vi "Measurement UI.vi"() -> ()   [LabVIEW 2021, in "adc_linearityMeasurement.lvlib"]
uses:
  adc_linearityMeasurement.lvlib
panel:
  in  "MeasGraphs":T1(tab)
  out "TimeDomain":waveform(dbl)(graph) caption="AC"
  out "Histogram":T2(graph) caption="TimeDomain 2"
  out "DNL waveform":dbl[](graph) caption="AC"
  out "INL waveform":dbl[](graph) caption="AC"
  out "Channel name":string
  out "Number of missing codes":i32
  out "Minimum hits position":i32
  out "Minimum hits per code":i32
  out "INL position":i32
  out "INL":dbl
  out "DNL position":i32
  out "DNL":dbl
  out "Histogram: h(x)":i32[](array[numeric])
  out "Histogram X":dbl[](array[numeric])
  out "Time domain":dbl[](array[numeric])
  out "dt":dbl
  in  "Digital capture resource name":string
  in  "Analog source resource name":string
  out "MeasTable":string[][](table)
  in  "MeasSettingsOptions":i32(listbox)
  in  "Digital capture":string="Digital capture"
  in  "Analog source":string="Analog source"
  in  "ADC parameters":string="ADC parameters"
  in  "MeasSettings":bool
  out "Samples to acquire":u32 caption="SAMPLES TO ACQUIRE"
  in  "Digital capture test duration":dbl=800000.0 caption="TEST DURATION" format="%#_6ps"
  in  "Triangle frequency":dbl=20.0 caption="FREQUENCY" format="%#_6pHz"
  in  "Triangle amplitude":dbl=5.1 caption="AMPLITUDE" format="%#_6pV"
  in  "Sine amplitude":dbl=5.1 caption="AMPLITUDE" format="%#_6pV"
  in  "Sine frequency":dbl=1000.0 caption="FREQUENCY" format="%#_6pHz"
  out "Input frequency":dbl caption="INPUT FREQUENCY" format="%#_6pHz"
  in  "Input channel":i32 caption="INPUT CHANNEL" min=0 max=100 step=1
  in  "Ramp amplitude":dbl=5.05 caption="RAMP AMPLITUDE" format="%#_6pV"
  in  "Ramp type":u32(ring) caption="RAMP TYPE" items=["Ascending", "Descending"]
  in  "Ramp duration":dbl=10.0 caption="RAMP DURATION" format="%#_6ps"
  in  "Full scale range":dbl=10.0 caption="FULL SCALE RANGE" format="%#_6pV"
  in  "Input signal":u32(ring) caption="INPUT  SIGNAL" items=["Sine", "Triangle", "Ramp"]
  in  "Digital capture sample rate":dbl=800000.0 caption="SAMPLE RATE" format="%#_6pS/s"
  in  "DSGresourcename":tag caption="RESOURCE NAME"
  in  "DPIresourcename":refnum<k15> caption="RESOURCE NAME"
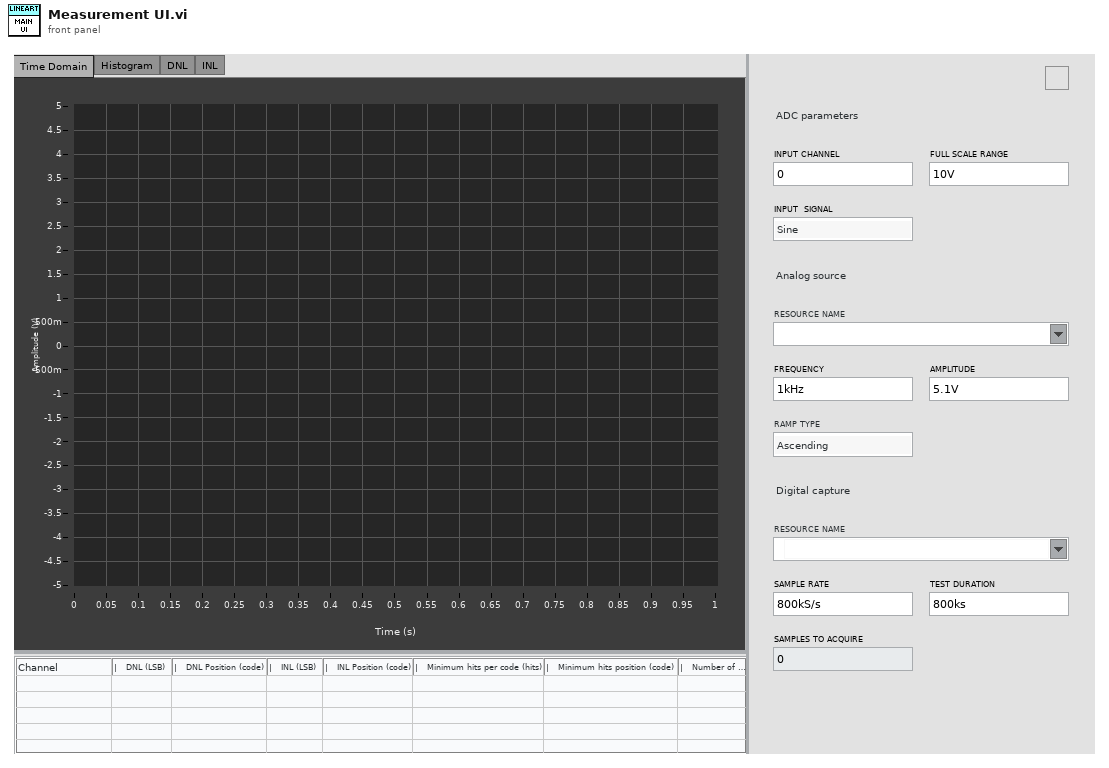
[diagram p1: front panel]
types:
  T1 = enum32{"Time Domain", "Histogram", "DNL", "INL", "Hiden controls"}
  T2 = cluster{"X Values":dbl[], "Histogram: h(x)":i32[]}
  T3 = enum16{"open", "replace", "create", "open or create", "replace or create", "replace or create with confirmation"}
  T4 = cluster{"Histogram X":dbl[], "Histogram: h(x)":i32[]}
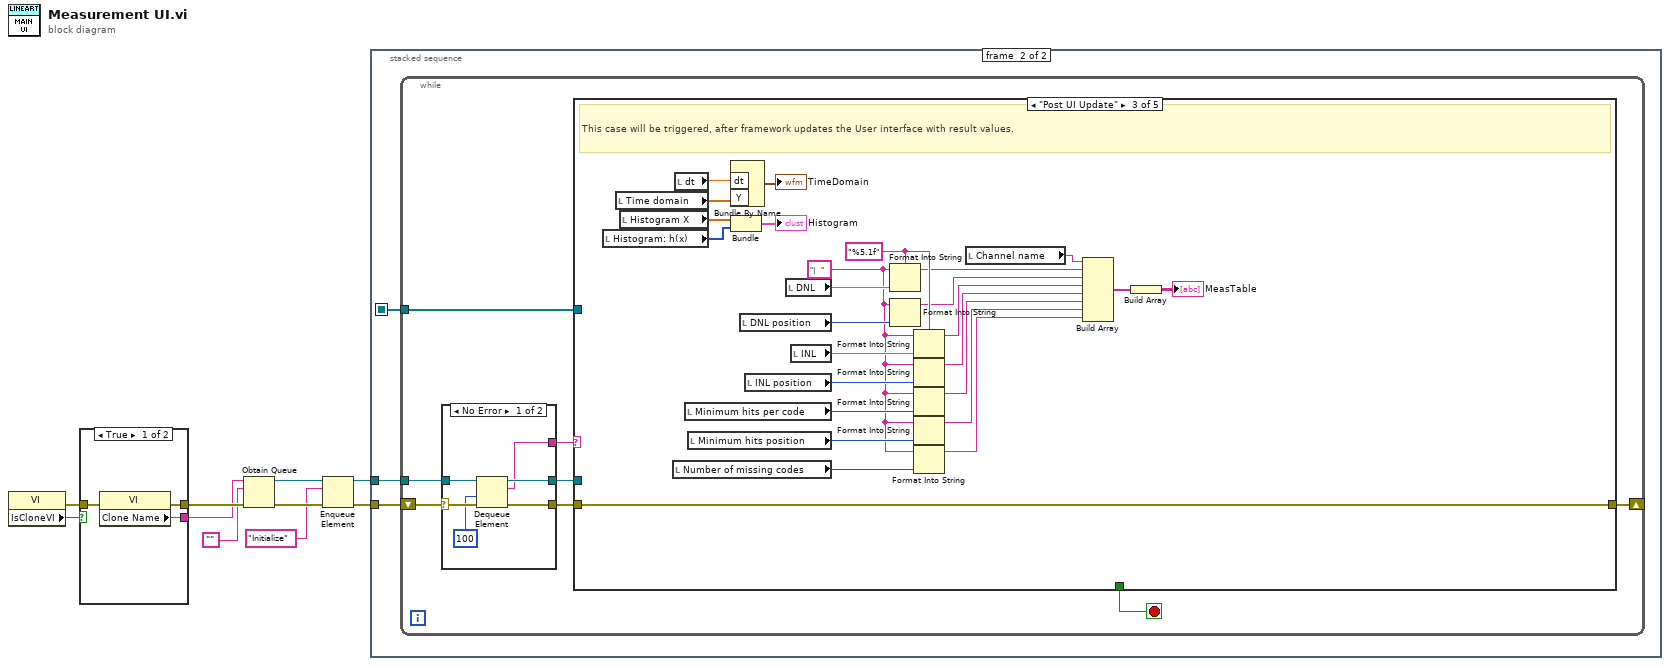
[diagram p0: block diagram]
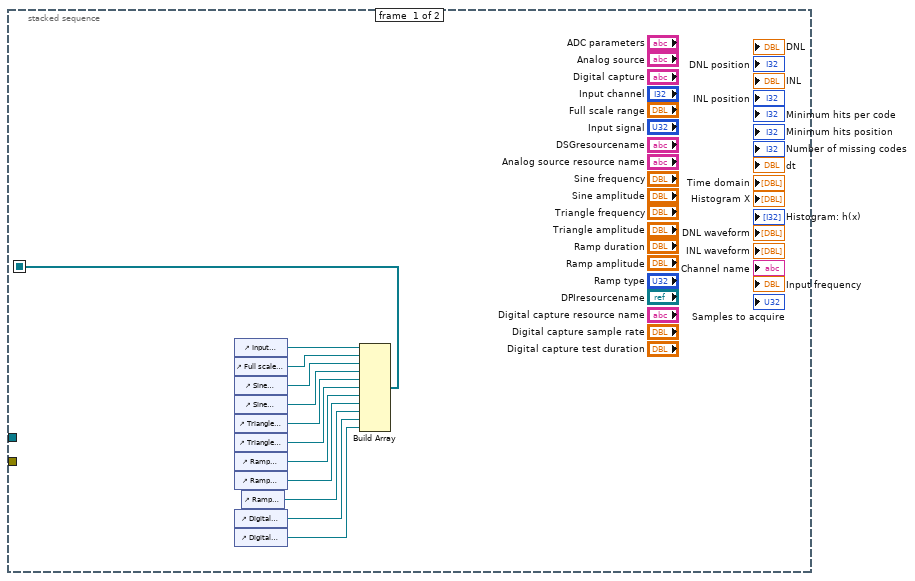
[diagram p2: hidden frame]
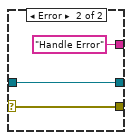
[diagram p3: hidden frame]
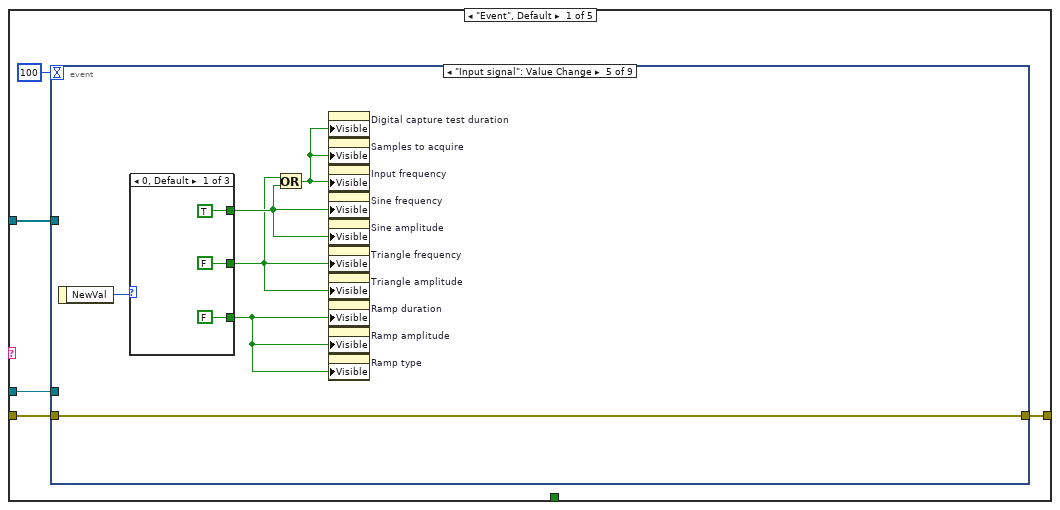
[diagram p4: hidden frame]
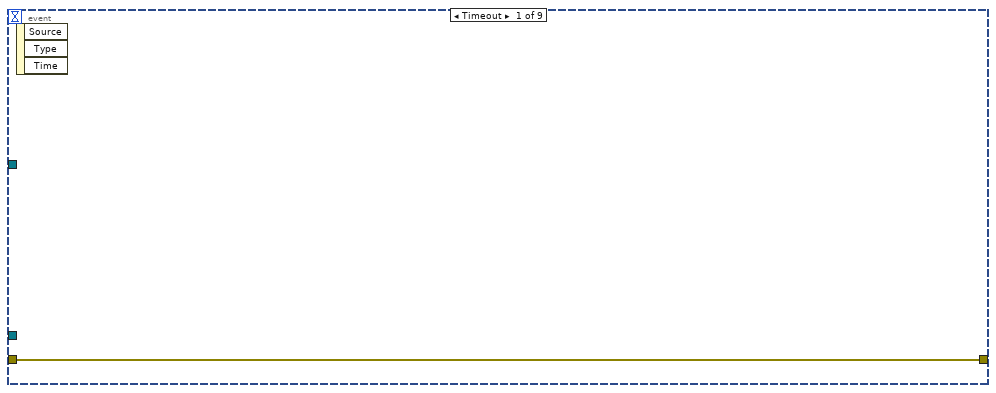
[diagram p5: hidden frame]
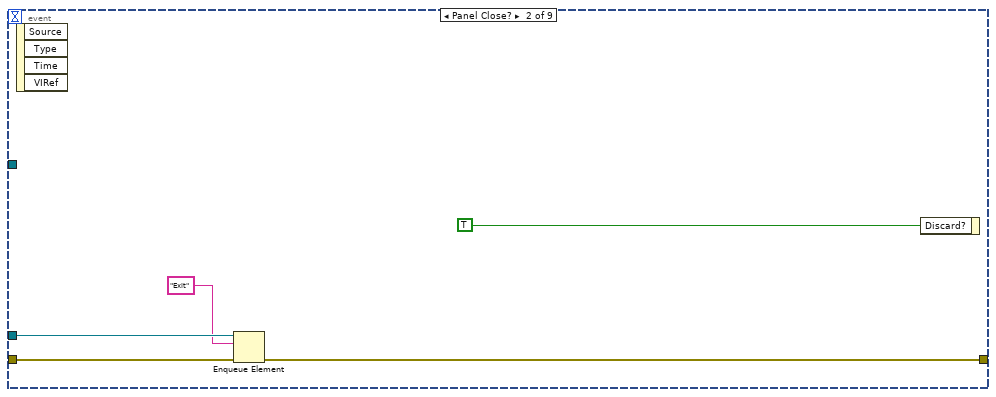
[diagram p6: hidden frame]
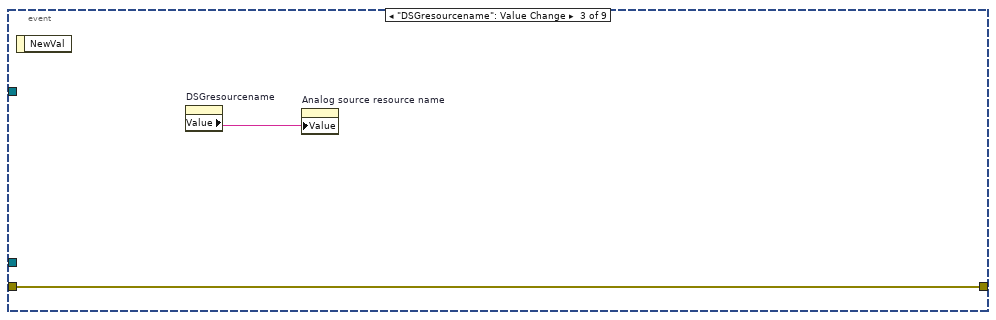
[diagram p7: hidden frame]
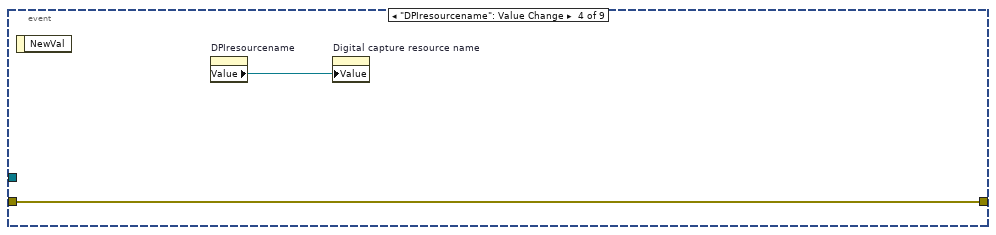
[diagram p8: hidden frame]
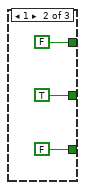
[diagram p9: hidden frame]
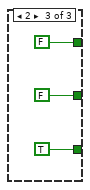
[diagram p10: hidden frame]
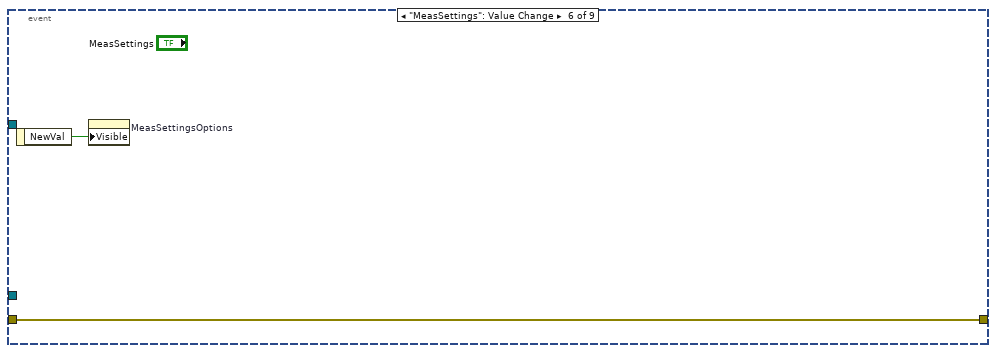
[diagram p11: hidden frame]
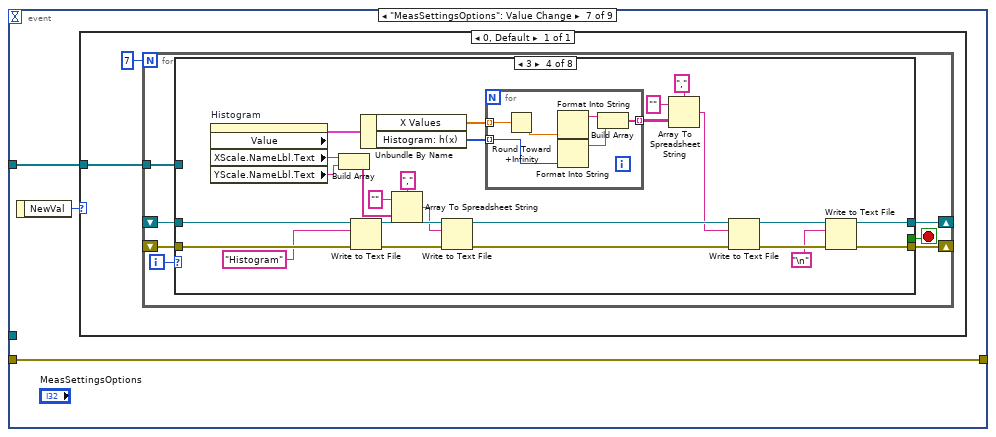
[diagram p12: hidden frame]
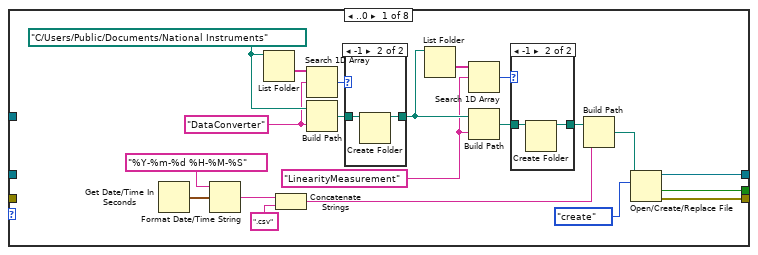
[diagram p13: hidden frame]
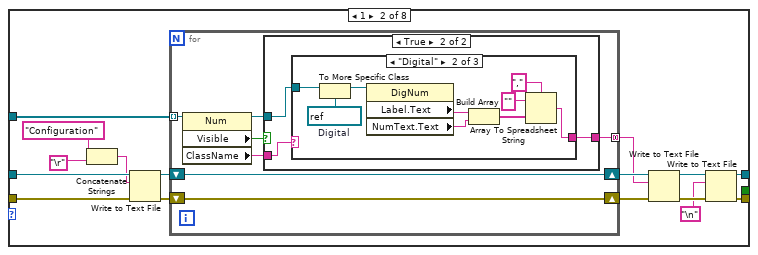
[diagram p16: hidden frame]
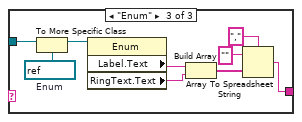
[diagram p19: hidden frame]
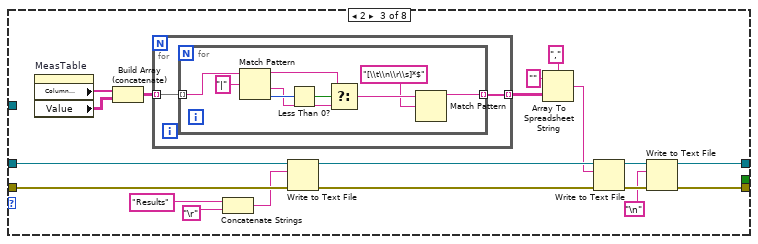
[diagram p20: hidden frame]
diagram:
  n1 = property class="VI"() -> (error out=w1:errorcluster, "IsCloneVI"=w2:bool)  [unwired: 2 in, 1 out]
  n2 = case shown="True" w2 {
    tunnel: [w13 w16] -> w10
    tunnel: [w12 w15] -> w9
    tunnel: w1 -> [w11 w14]
    frame True {
      n3 = property class="VI"(error in=w11) -> (error out=w13:errorcluster, "Clone Name"=w12:string)  [unwired: 1 in, 1 out]
    }
    frame False {
      n4 = property class="VI"(error in=w14) -> (error out=w16:errorcluster, "Name"=w15:string)  [unwired: 1 in, 1 out]
    }
  }
  n5 = Obtain Queue(name (unnamed)=w9, element data type="", error in (no error)=w10) -> (queue out=w6:refnum<queue>, error out=w8:errorcluster)  [unwired: 2 in, 1 out]
  n6 = Enqueue Element(queue=w6, element="Initialize", error in (no error)=w8) -> (queue out=w5:refnum<queue>, error out=w7:errorcluster)  [unwired: 1 in, 1 out]
  n7 = stacked-sequence {
    seq-local: [w17 _] -> [_ w29]
    tunnel: w7 -> [_ w31]
    tunnel: w5 -> [_ w30]
    frame #0 {
      n8 = control-ref of="Input channel"() -> (w28:refnum<vi>)
      n9 = control-ref of="Full scale range"() -> (w27:refnum<vi>)
      n10 = control-ref of="Sine frequency"() -> (w26:refnum<vi>)
      n11 = control-ref of="Sine amplitude"() -> (w25:refnum<vi>)
      n12 = control-ref of="Triangle frequency"() -> (w24:refnum<vi>)
      n13 = control-ref of="Triangle amplitude"() -> (w23:refnum<vi>)
      n14 = control-ref of="Ramp duration"() -> (w22:refnum<vi>)
      n15 = control-ref of="Ramp amplitude"() -> (w21:refnum<vi>)
      n16 = control-ref of="Digital capture sample rate"() -> (w19:refnum<vi>)
      n17 = control-ref of="Digital capture test duration"() -> (w18:refnum<vi>)
      n18 = control-ref of="Ramp type"() -> (w20:refnum<vi>)
      n19 = Build Array(w28, w27, w26, w25, w24, w23, w22, w21, w20, w19, w18) -> (w17:refnum<vi>[])
    }
    frame #1 {
      n20 = while {
        shift-right: [w34] -> _
        shift-left: w31 -> [w39]
        tunnel: w30 -> [w37]
        tunnel: w29 -> [w32]
        stop <- w33 stop-if-true
        n21 = case shown="No Error" w39 {
          selector: w39 -> [w45 w48]
          tunnel: [w44 w48] -> w38
          tunnel: w37 -> [w43 w47]
          tunnel: [w42 w47] -> w36
          tunnel: [w41 "Handle Error"] -> w35
          frame No Error {
            n22 = Dequeue Element(queue=w43, timeout in ms (-1)=100, error in (no error)=w45) -> (queue out=w42:refnum<queue>, element=w41:string, error out=w44:errorcluster)  [unwired: 1 out]
          }
          frame Error {
          }
        }
        n23 = case shown="\"Post UI Update\"" w35 {
          tunnel: w38 -> [w52 w315 w343 w350 w351]
          tunnel: w36 -> [w50 _ _ w348 _]
          tunnel: [w53 w315 w343 w345 w351] -> w34
          tunnel: [_ _ _ TRUE _] -> w33
          tunnel: w32 -> [w49 _ _ _ _]
          frame "Event", Default {
            n24 = event shown="[4] \"Input signal\": Value Change" {
              selector: _ -> [_ _ _ _ _ _ _ _ _]
              dyn-events: _ -> [_ _ _ _ _ _ _ _ _]
              timeout: 100 -> [_ _ _ _ _ _ _ _ _]
              tunnel: [w54 w57 w60 w62 w64 w80 w82 w292 w293] -> w53
              tunnel: w52 -> [w54 w58 w60 w62 w64 w80 w82 w292 w293]
              tunnel: w50 -> [_ w56 _ _ _ _ _ _ _]
              tunnel: w49 -> [_ _ _ _ _ _ w81 _ _]
              event Timeout {
                n25 = event-data() -> ()  [unwired: 1 in, 3 out]
              }
              event Panel Close? {
                n26 = event-data() -> ()  [unwired: 1 in, 4 out]
                n27 = Enqueue Element(queue=w56, element="Exit", error in (no error)=w58) -> (error out=w57:errorcluster)  [unwired: 1 in, 2 out]
                n28 = event-data("Discard?"=TRUE) -> ()  [unwired: 1 in, 1 out]
              }
              event "DSGresourcename": Value Change {
                n29 = event-data() -> ()  [unwired: 1 in, 1 out]
                n30 = property on="DSGresourcename" class="DAQmxName"() -> ("Value"=w61:string)  [unwired: 2 in, 2 out]
                n31 = property on="Analog source resource name" class="Str"("Value"=w61) -> ()  [unwired: 2 in, 2 out]
              }
              event "DPIresourcename": Value Change {
                n32 = event-data() -> ()  [unwired: 1 in, 1 out]
                n33 = property on="DPIresourcename" class="IVIName"() -> ("Value"=w63:refnum<k15>)  [unwired: 2 in, 2 out]
                n34 = property on="Digital capture resource name" class="Str"("Value"=w63) -> ()  [unwired: 2 in, 2 out]
              }
              event "Input signal": Value Change {
                n35 = event-data() -> ("NewVal"=w69:u32)  [unwired: 1 in]
                n36 = case shown="0, Default" w69 {
                  tunnel: [TRUE FALSE FALSE] -> w67
                  tunnel: [FALSE TRUE FALSE] -> w66
                  tunnel: [FALSE FALSE TRUE] -> w68
                  frame 0, Default {
                  }
                  frame 1 {
                  }
                  frame 2 {
                  }
                }
                n37 = Or(x=w66, y=w67) -> (x .or. y?=w65:bool)
                n38 = property on="Digital capture test duration" class="DigNum (strict)"("Visible"=w65) -> ()  [unwired: 2 in, 2 out]
                n39 = property on="Samples to acquire" class="DigNum (strict)"("Visible"=w65) -> ()  [unwired: 2 in, 2 out]
                n40 = property on="Input frequency" class="DigNum (strict)"("Visible"=w65) -> ()  [unwired: 2 in, 2 out]
                n41 = property on="Sine frequency" class="DigNum (strict)"("Visible"=w67) -> ()  [unwired: 2 in, 2 out]
                n42 = property on="Sine amplitude" class="DigNum (strict)"("Visible"=w67) -> ()  [unwired: 2 in, 2 out]
                n43 = property on="Triangle frequency" class="DigNum (strict)"("Visible"=w66) -> ()  [unwired: 2 in, 2 out]
                n44 = property on="Triangle amplitude" class="DigNum (strict)"("Visible"=w66) -> ()  [unwired: 2 in, 2 out]
                n45 = property on="Ramp duration" class="DigNum (strict)"("Visible"=w68) -> ()  [unwired: 2 in, 2 out]
                n46 = property on="Ramp amplitude" class="DigNum (strict)"("Visible"=w68) -> ()  [unwired: 2 in, 2 out]
                n47 = property on="Ramp type" class="Ring (strict)"("Visible"=w68) -> ()  [unwired: 2 in, 2 out]
              }
              event "MeasSettings": Value Change {
                n48 = event-data() -> ("NewVal"=w79:bool)  [unwired: 1 in]
                n49 = property on="MeasSettingsOptions" class="LstBox (strict)"("Visible"=w79) -> ()  [unwired: 2 in, 2 out]
              }
              event "MeasSettingsOptions": Value Change {
                n50 = event-data() -> ("NewVal"=w83:i32)  [unwired: 1 in]
                n51 = case shown="0, Default" w83 {
                  tunnel: w81 -> [w85]
                  frame 0, Default {
                    n52 = for {
                      N: 7 -> [_]
                      shift-right: [w90] -> _
                      shift-left: _ -> [w89]
                      shift-right: [w88] -> _
                      shift-left: _ -> [w87]
                      tunnel: w85 -> [w86]
                      i -> [w92]
                      stop <- w91 stop-if-true
                      n53 = case shown="3" w92 {
                        tunnel: [w106 _ _ _ _ _ _ _] -> w91
                        tunnel: [w112 w123 w169 w197 w228 w261 refnum<file> refnum ("refnum out") w288] -> w90
                        tunnel: w89 -> [_ w134 w182 w218 w247 w273 w283 w288]
                        tunnel: [w105 w122 w168 w195 w226 w260 w281 w287] -> w88
                        tunnel: w87 -> [_ w132 w181 w217 w246 w272 w282 w287]
                        tunnel: w86 -> [_ w120 _ _ _ _ _ _]
                        frame ..0 {
                          w101 = "LinearityMeasurement" ("prompt")
                          w108 = "DataConverter" ("prompt")
                          w111 = path "C:/Users/Public/Documents/National Instruments" ("base path")
                          n54 = Get Date/Time In Seconds() -> (seconds since 1Jan1904=w98:timestamp)
                          n55 = Format Date/Time String(time format string (%c)="%Y-%m-%d %H-%M-%S", seconds (now)=w98) -> (date/time string=w97:string)  [unwired: 1 in]
                          n56 = List Folder(path=w111) -> (folder names=w109:string[])  [unwired: 3 in, 3 out]
                          n57 = Concatenate Strings(w97, ".csv" ("string")) -> (w94:string)
                          n58 = Search 1D Array(1D array=w109, element=w108) -> (index of element=w107:i32)  [unwired: 1 in]
                          n59 = Build Path(base path=w111, name or relative path=w108) -> (appended path=w110:path)
                          n60 = case shown="-1" w107 {
                            tunnel: w110 -> [w117 w119]
                            tunnel: [w117 w118] -> w102
                            frame Default {
                            }
                            frame -1 {
                              n61 = Create Folder(path (use dialog)=w119) -> (created path=w118:path)  [unwired: 2 in, 2 out]
                            }
                          }
                          n62 = List Folder(path=w102) -> (folder names=w104:string[])  [unwired: 3 in, 3 out]
                          n63 = Search 1D Array(1D array=w104, element=w101) -> (index of element=w103:i32)  [unwired: 1 in]
                          n64 = Build Path(base path=w102, name or relative path=w101) -> (appended path=w100:path)
                          n65 = case shown="-1" w103 {
                            tunnel: w100 -> [w114 w116]
                            tunnel: [w114 w115] -> w95
                            frame Default {
                            }
                            frame -1 {
                              n66 = Create Folder(path (use dialog)=w116) -> (created path=w115:path)  [unwired: 2 in, 2 out]
                            }
                          }
                          n67 = Build Path(base path=w95, name or relative path=w94) -> (appended path=w93:path)
                          n68 = Open/Create/Replace File(file path (use dialog)=w93, operation (0:open)=T3."create") -> (refnum out=w112:refnum<file>, cancelled=w106:bool, error out=w105:errorcluster)  [unwired: 4 in]
                        }
                        frame 1 {
                          n69 = Concatenate Strings("Configuration" ("format string"), "\r") -> (w129:string)
                          n70 = Write to Text File(file (use dialog)=w134, text=w129, error in=w132) -> (refnum out=w135:refnum<file>, error out=w133:errorcluster)  [unwired: 1 in, 1 out]
                          n71 = for {
                            tunnel: w120 -> [w138] mode=indexing
                            shift-right: [w142] -> w128
                            shift-left: w135 -> [w142]
                            shift-right: [w141] -> w126
                            shift-left: w133 -> [w141]
                            tunnel: [w140] -> w124 mode=concatenating
                            n72 = property class="Num"(reference=w138) -> (reference out=w139:refnum<vi>, "Visible"=w137:bool, "ClassName"=w136:string)  [unwired: 1 in, 1 out]
                            n73 = case shown="True" w137 {
                              tunnel: [_ w145] -> w140
                              tunnel: w139 -> [_ w144]
                              tunnel: w136 -> [_ w143]
                              frame False {
                              }
                              frame True {
                                n74 = case shown="\"Digital\"" w143 {
                                tunnel: [_ w149 w158] -> w145
                                tunnel: w144 -> [_ w147 w156]
                                frame Default {
                                }
                                frame "Digital" {
                                w146 = refnum<vi> refnum  # Digital
                                n75 = To More Specific Class(target class=w146, reference=w147) -> (specific class reference=w148:refnum<vi>)  [unwired: 1 in, 1 out]
                                n76 = property class="DigNum"(reference=w148) -> ("Label.Text"=w154:string, "NumText.Text"=w153:string)  [unwired: 1 in, 2 out]
                                n77 = Build Array(w154, w153) -> (w150:string[])
                                n78 = Array To Spreadsheet String(delimiter (Tab)=",", array=w150, 3:"" ("format string")) -> (spreadsheet string=w149:string)
                                }
                                frame "Enum" {
                                w155 = refnum<vi> refnum  # Enum
                                n79 = To More Specific Class(target class=w155, reference=w156) -> (specific class reference=w157:refnum<vi>)  [unwired: 1 in, 1 out]
                                n80 = property class="Enum"(reference=w157) -> ("Label.Text"=w163:string, "RingText.Text"=w162:string)  [unwired: 1 in, 2 out]
                                n81 = Build Array(w163, w162) -> (w159:string[])
                                n82 = Array To Spreadsheet String(delimiter (Tab)=",", array=w159, 3:"" ("format string")) -> (spreadsheet string=w158:string)
                                }
                                }
                              }
                            }
                          }
                          n83 = Write to Text File(file (use dialog)=w128, text=w124, error in=w126) -> (refnum out=w127:refnum<file>, error out=w125:errorcluster)  [unwired: 1 in, 1 out]
                          n84 = Write to Text File(file (use dialog)=w127, text="\n", error in=w125) -> (refnum out=w123:refnum<file>, error out=w122:errorcluster)  [unwired: 1 in, 1 out]
                        }
                        frame 2 {
                          n85 = property on="MeasTable" class="Tbl (strict)"() -> ("Column Headers[]"=w179:string[], "Value"=w178:string[][])  [unwired: 2 in, 2 out]
                          n86 = Build Array (concatenate)(w179, w178) -> (w177:string[][])
                          n87 = for {
                            tunnel: w177 -> [w184] mode=indexing
                            tunnel: [w183] -> w176 mode=indexing
                            n88 = for {
                              tunnel: w184 -> [w186] mode=indexing
                              tunnel: [w185] -> w183 mode=indexing
                              n89 = Match Pattern(string=w186, regular expression="|") -> (before substring=w190:string, after substring=w189:string, offset past match=w192:i32)  [unwired: 1 in, 1 out]
                              n90 = Less Than 0?(x=w192) -> (x < 0?=w191:bool)
                              n91 = Select(t=w190, s=w191, f=w189) -> (s? t:f=w188:string)
                              n92 = Match Pattern(string=w188, regular expression="[\\t\\n\\r\\s]*$") -> (before substring=w185:string)  [unwired: 1 in, 3 out]
                            }
                          }
                          n93 = Concatenate Strings("Results" ("element"), "\r") -> (w164:string)
                          n94 = Write to Text File(file (use dialog)=w182, text=w164, error in=w181) -> (refnum out=w180:refnum<file>, error out=w172:errorcluster)  [unwired: 1 in, 1 out]
                          n95 = Array To Spreadsheet String(delimiter (Tab)=",", array=w176, 3:"" ("format string")) -> (spreadsheet string=w173:string)
                          n96 = Write to Text File(file (use dialog)=w180, text=w173, error in=w172) -> (refnum out=w171:refnum<file>, error out=w170:errorcluster)  [unwired: 1 in, 1 out]
                          n97 = Write to Text File(file (use dialog)=w171, text="\n", error in=w170) -> (refnum out=w169:refnum<file>, error out=w168:errorcluster)  [unwired: 1 in, 1 out]
                        }
                        frame 3 {
                          n98 = property on="Histogram" class="XYGraph (strict)"() -> ("Value"=w201:T2, "XScale.NameLbl.Text"=w216:string, "YScale.NameLbl.Text"=w215:string)  [unwired: 2 in, 2 out]
                          n99 = Build Array(w216, w215) -> (w214:string[])
                          n100 = Write to Text File(file (use dialog)=w218, text="Histogram" ("string"), error in=w217) -> (refnum out=w211:refnum<file>, error out=w210:errorcluster)  [unwired: 1 in, 1 out]
                          n101 = Unbundle By Name(w201) -> ("X Values"=w202:dbl[], "Histogram: h(x)"=w203:i32[])
                          n102 = Array To Spreadsheet String(delimiter (Tab)=",", array=w214, 3:"" ("format string")) -> (spreadsheet string=w209:string)
                          n103 = Write to Text File(file (use dialog)=w211, text=w209, error in=w210) -> (refnum out=w208:refnum<file>, error out=w207:errorcluster)  [unwired: 1 in, 1 out]
                          n104 = for {
                            tunnel: w202 -> [w221] mode=indexing
                            tunnel: w203 -> [w220] mode=indexing
                            tunnel: [w222] -> w204 mode=indexing
                            n105 = Round Toward +Infinity(x=w221) -> (ceil(x): smallest int >= x=w219:dbl)
                            n106 = Format Into String(w219) -> (resulting string=w223:string)  [unwired: 3 in, 1 out]
                            n107 = Format Into String(w220) -> (resulting string=w224:string)  [unwired: 3 in, 1 out]
                            n108 = Build Array(w223, w224) -> (w222:string[])
                          }
                          n109 = Array To Spreadsheet String(delimiter (Tab)=",", array=w204, 3:"" ("format string")) -> (spreadsheet string=w200:string)
                          n110 = Write to Text File(file (use dialog)=w208, text=w200, error in=w207) -> (refnum out=w198:refnum<file>, error out=w196:errorcluster)  [unwired: 1 in, 1 out]
                          n111 = Write to Text File(file (use dialog)=w198, text="\n", error in=w196) -> (refnum out=w197:refnum<file>, error out=w195:errorcluster)  [unwired: 1 in, 1 out]
                        }
                        frame 4 {
                          n112 = property on="DNL waveform" class="WFGraph (strict)"() -> ("Value"=w231:dbl[], "XScale.NameLbl.Text"=w245:string, "YScale.NameLbl.Text"=w244:string)  [unwired: 2 in, 2 out]
                          n113 = Build Array(w245, w244) -> (w243:string[])
                          n114 = Write to Text File(file (use dialog)=w247, text="DNL" ("string"), error in=w246) -> (refnum out=w240:refnum<file>, error out=w239:errorcluster)  [unwired: 1 in, 1 out]
                          n115 = Array To Spreadsheet String(delimiter (Tab)=",", array=w243, 3:"" ("format string")) -> (spreadsheet string=w238:string)
                          n116 = for {
                            tunnel: w231 -> [w252] mode=indexing
                            tunnel: [w253] -> w233 mode=indexing
                            i -> [w251]
                            n117 = Increment(x=w251) -> (x+1=w248:i32)
                            n118 = Format Into String(w252) -> (resulting string=w249:string)  [unwired: 3 in, 1 out]
                            n119 = Format Into String(w248) -> (resulting string=w250:string)  [unwired: 3 in, 1 out]
                            n120 = Build Array(w250, w249) -> (w253:string[])
                          }
                          n121 = Write to Text File(file (use dialog)=w240, text=w238, error in=w239) -> (refnum out=w237:refnum<file>, error out=w236:errorcluster)  [unwired: 1 in, 1 out]
                          n122 = Array To Spreadsheet String(delimiter (Tab)=",", array=w233, 3:"" ("format string")) -> (spreadsheet string=w232:string)
                          n123 = Write to Text File(file (use dialog)=w237, text=w232, error in=w236) -> (refnum out=w229:refnum<file>, error out=w227:errorcluster)  [unwired: 1 in, 1 out]
                          n124 = Write to Text File(file (use dialog)=w229, text="\n", error in=w227) -> (refnum out=w228:refnum<file>, error out=w226:errorcluster)  [unwired: 1 in, 1 out]
                        }
                        frame 5 {
                          n125 = property on="INL waveform" class="WFGraph (strict)"() -> ("Value"=w255:dbl[], "XScale.NameLbl.Text"=w271:string, "YScale.NameLbl.Text"=w270:string)  [unwired: 2 in, 2 out]
                          n126 = Build Array(w271, w270) -> (w269:string[])
                          n127 = Write to Text File(file (use dialog)=w273, text="INL" ("string"), error in=w272) -> (refnum out=w266:refnum<file>, error out=w265:errorcluster)  [unwired: 1 in, 1 out]
                          n128 = Array To Spreadsheet String(delimiter (Tab)=",", array=w269, 3:"" ("format string")) -> (spreadsheet string=w264:string)
                          n129 = for {
                            tunnel: w255 -> [w277] mode=indexing
                            tunnel: [w278] -> w257 mode=indexing
                            i -> [w276]
                            n130 = Increment(x=w276) -> (x+1=w274:i32)
                            n131 = Format Into String(w277) -> (resulting string=w275:string)  [unwired: 3 in, 1 out]
                            n132 = Format Into String(w274) -> (resulting string=w279:string)  [unwired: 3 in, 1 out]
                            n133 = Build Array(w279, w275) -> (w278:string[])
                          }
                          n134 = Write to Text File(file (use dialog)=w266, text=w264, error in=w265) -> (refnum out=w263:refnum<file>, error out=w262:errorcluster)  [unwired: 1 in, 1 out]
                          n135 = Array To Spreadsheet String(delimiter (Tab)=",", array=w257, 3:"" ("format string")) -> (spreadsheet string=w256:string)
                          n136 = Write to Text File(file (use dialog)=w263, text=w256, error in=w262) -> (refnum out=w261:refnum<file>, error out=w260:errorcluster)  [unwired: 1 in, 1 out]
                        }
                        frame 6 {
                          w285 = FALSE ("Visible")
                          n137 = Close File(refnum=w283, error in=w282) -> (error out=w281:errorcluster)  [unwired: 1 out]
                          n138 = property on="MeasSettingsOptions" class="LstBox (strict)"("Visible"=w285, "Value"=-1 ("MeasSettingsOptions")) -> (error out=w286:errorcluster)  [unwired: 2 in, 1 out]
                          n139 = property on="MeasSettings" class="Bool (strict)"(error in=w286, "Value"=w285) -> ()  [unwired: 1 in, 2 out]
                        }
                        frame Default {
                        }
                      }
                    }
                  }
                }
              }
              event Mouse Down {
                w290 = FALSE ("Visible")
                n140 = event-data() -> ()  [unwired: 1 in, 1 out]
                n141 = property on="MeasSettingsOptions" class="LstBox (strict)"("Visible"=w290, "Value"=-1 ("MeasSettingsOptions")) -> (error out=w291:errorcluster)  [unwired: 2 in, 1 out]
                n142 = property on="MeasSettings" class="Bool (strict)"(error in=w291, "Value"=w290) -> ()  [unwired: 1 in, 2 out]
              }
              event "INL waveform", "DNL waveform", "Histogram", "TimeDomain": Shortcut Menu Selection (User) {
                n143 = event-data() -> ("ItemTag"=w297:string)  [unwired: 1 in]
                n144 = case shown="\"INL\"" "MeasGraphs" {
                  tunnel: [w298 w299 w300 w301] -> w295
                  frame "Time Domain", Default {
                    n145 = control-ref of="TimeDomain"() -> (w298:refnum<vi>)
                  }
                  frame "Histogram" {
                    n146 = control-ref of="Histogram"() -> (w299:refnum<vi>)
                  }
                  frame "DNL" {
                    n147 = control-ref of="DNL waveform"() -> (w300:refnum<vi>)
                  }
                  frame "INL" {
                    n148 = control-ref of="INL waveform"() -> (w301:refnum<vi>)
                  }
                }
                n149 = case shown="\"ZOOM_TO_RECTANGLE\", Default" w297 {
                  tunnel: [2 ("Palette:Active Tool") 3 ("Palette:Active Tool") 4 ("Palette:Active Tool") 5 ("Palette:Active Tool") 1 ("Palette:Active Tool")] -> w294
                  frame "ZOOM_TO_RECTANGLE", Default {
                  }
                  frame "X_ZOOM" {
                  }
                  frame "Y_ZOOM" {
                  }
                  frame "ZOOM_TO_FIT" {
                  }
                  frame "PANNING_TOOL" {
                  }
                }
                n150 = property class="WFGraph"(reference=w295, "ActPaletteTool"=w294) -> ()  [unwired: 1 in, 2 out]
              }
            }
          }
          frame "Initialize" {
            w307 = 2 ("Palette:Active Tool")
            w311 = string[] ["Export data"] ("Item Names")
            w314 = "<Select Device>"
            n151 = property on="TimeDomain" class="WFGraph (strict)"("ActPaletteTool"=w307) -> ()  [unwired: 2 in, 2 out]
            n152 = property on="Histogram" class="XYGraph (strict)"("ActPaletteTool"=w307) -> ()  [unwired: 2 in, 2 out]
            n153 = property on="DSGresourcename" class="DAQmxName"("Value"=w314) -> ()  [unwired: 2 in, 2 out]
            n154 = property on="DPIresourcename" class="IVIName"("Value"=w314) -> ()  [unwired: 2 in, 2 out]
            n155 = property on="DNL waveform" class="WFGraph (strict)"("ActPaletteTool"=w307) -> ()  [unwired: 2 in, 2 out]
            n156 = property on="MeasGraphs" class="TabCtl (strict)"("Value"=T1."Histogram" ("MeasGraphs")) -> ()  [unwired: 2 in, 2 out]
            n157 = property on="Input signal" class="Ring (strict)"("Val(Sgnl)"=enum16{"Sine", "Triangle", "Ramp"}."Sine" ("Value (Signaling)")) -> ()  [unwired: 2 in, 2 out]
            n158 = property on="INL waveform" class="WFGraph (strict)"("ActPaletteTool"=w307) -> ()  [unwired: 2 in, 2 out]
            n159 = property on="MeasSettingsOptions" class="LstBox (strict)"("Item Names"=w311, "Value"=-1 ("MeasSettingsOptions"), "Visible"=FALSE, "Disabled Items"=i32[] []) -> ()  [unwired: 2 in, 2 out]
            n160 = for {
              tunnel: w311 -> [_] mode=indexing
              i -> [w317]
              n161 = property on="MeasSettingsOptions" class="LstBox (strict)"("Active Row"=w317, "Cell Height"=30 ("Active Row:Cell Height")) -> ()  [unwired: 2 in, 2 out]
            }
          }
          frame "Post UI Update" {
            w320 = "|   " ("initial string")
            w333 = "%5.1f" ("format string")
            # "This case will be triggered, after framework updates the User interface with result values."
            n162 = local read "Histogram: h(x)"() -> (w338:i32[])
            n163 = local read "Time domain"() -> (w341:dbl[])
            n164 = local read "Histogram X"() -> (w339:dbl[])
            n165 = local read "Number of missing codes"() -> (w319:i32)
            n166 = local read "dt"() -> (w342:dbl)
            n167 = local read "Minimum hits per code"() -> (w331:i32)
            n168 = local read "Minimum hits position"() -> (w330:i32)
            n169 = Bundle By Name("dt"=w342, "Y"=w341) -> (→"TimeDomain":waveform(dbl))  [unwired: 1 in]
            n170 = Bundle("Histogram X"=w339, "Histogram: h(x)"=w338) -> (→"Histogram":T4)  [unwired: 1 in]
            n171 = local read "DNL position"() -> (w335:i32)
            n172 = local read "INL position"() -> (w332:i32)
            n173 = local read "DNL"() -> (w336:dbl)
            n174 = local read "INL"() -> (w334:dbl)
            n175 = Format Into String(format string=w333, initial string=w320, w336) -> (resulting string=w329:string)  [unwired: 1 in, 1 out]
            n176 = Format Into String(initial string=w320, w335) -> (resulting string=w328:string)  [unwired: 2 in, 1 out]
            n177 = Format Into String(format string=w333, initial string=w320, w334) -> (resulting string=w327:string)  [unwired: 1 in, 1 out]
            n178 = Format Into String(initial string=w320, w332) -> (resulting string=w326:string)  [unwired: 2 in, 1 out]
            n179 = Format Into String(initial string=w320, w331) -> (resulting string=w325:string)  [unwired: 2 in, 1 out]
            n180 = Format Into String(initial string=w320, w330) -> (resulting string=w324:string)  [unwired: 2 in, 1 out]
            n181 = Format Into String(initial string=w320, w319) -> (resulting string=w318:string)  [unwired: 2 in, 1 out]
            n182 = local read "Channel name"() -> (w321:string)
            n183 = Build Array(w321, w329, w328, w327, w326, w325, w324, w318) -> (w323:string[])
            n184 = Build Array(w323) -> (→"MeasTable":string[][])
          }
          frame "Exit" {
            # "This case is triggered to close the User Interface from framework"
            n185 = Flush Queue(queue=w348, error in (no error)=w350) -> (queue out=w347:refnum<queue>, error out=w346:errorcluster)  [unwired: 1 out]
            n186 = Release Queue(queue=w347, force destroy? (F)=TRUE, error in (no error)=w346) -> (error out=w345:errorcluster)  [unwired: 2 out]
          }
          frame "Handle Error" {
          }
        }
      }
    }
  }
